vi "ResultsColumn.vi"(0 "Table Builder (Eingang)":refnum<class "Table Builder.lvclass">, 1 "Results out":T4={"Results"=[], "ResultPictures"={"Yes Ctl Refnum"=refnum, "No Ctl Refnum"=refnum}, "use Pictures"=FALSE, "Image Scale (%)"=100.0, "Autoscale? (T)"=TRUE, "Horizontal Align"=3, "Position"=0} {"Position" items=["First", "Last"]; "Horizontal Align" items=["Center", "Justified", "JustifiedAll", "Left", "Right"]}, 2 "empty?":bool, 3 "Font (Eingang)":refnum<class "Font.lvclass">, 5 "Row Formatting in":refnum<class "Formatting.lvclass">[](array[class]), 9 "Horizontal Align":i32, 11 "Fehler (Eingang, kein Fehler)":errorcluster, 12 "Result Cell Configuration":T1 {"Cell Defaults"."Vertical Align" items=["Bottom", "Middle", "Top"]; "Cell Defaults"."Horizontal Align" items=["Center", "Justified", "JustifiedAll", "Left", "Right"]}, 13 "BackgroundColor":u32, 14 "RowIndex":i32) -> (4 "Table Builder (Ausgang)":refnum<class "Table Builder.lvclass">, 6 "Row Formatting Array out":refnum<class "Formatting.lvclass">[](array[class]), 15 "Fehler (Ausgang)":errorcluster)   [LabVIEW 2020, in "PDF Interface.lvlib" / "PDF Interface Helper.lvlib"]
uses:
  PDF Interface Helper.lvlib
  <vilib>/Simplicity AI/SAI_PDF_API/Classes/Table Formatting/Formatting.lvclass
  <vilib>/Simplicity AI/SAI_PDF_API/Classes/Font/Font.lvclass
  PDFResults.ctl
  PDFResultPictures.ctl
  <vilib>/Simplicity AI/SAI_PDF_API/Classes/Table Builder/Controls/SAI_PDF_Cell Configuration.ctl
  <vilib>/Simplicity AI/SAI_PDF_API/Classes/Table Builder/Controls/SAI_PDF_Default Cell Format.ctl
  <vilib>/Simplicity AI/SAI_PDF_API/Classes/Table Builder/Controls/SAI_PDF_BorderLine.ctl
  <vilib>/Simplicity AI/SAI_PDF_API/Classes/Table Builder/Table Builder.lvclass
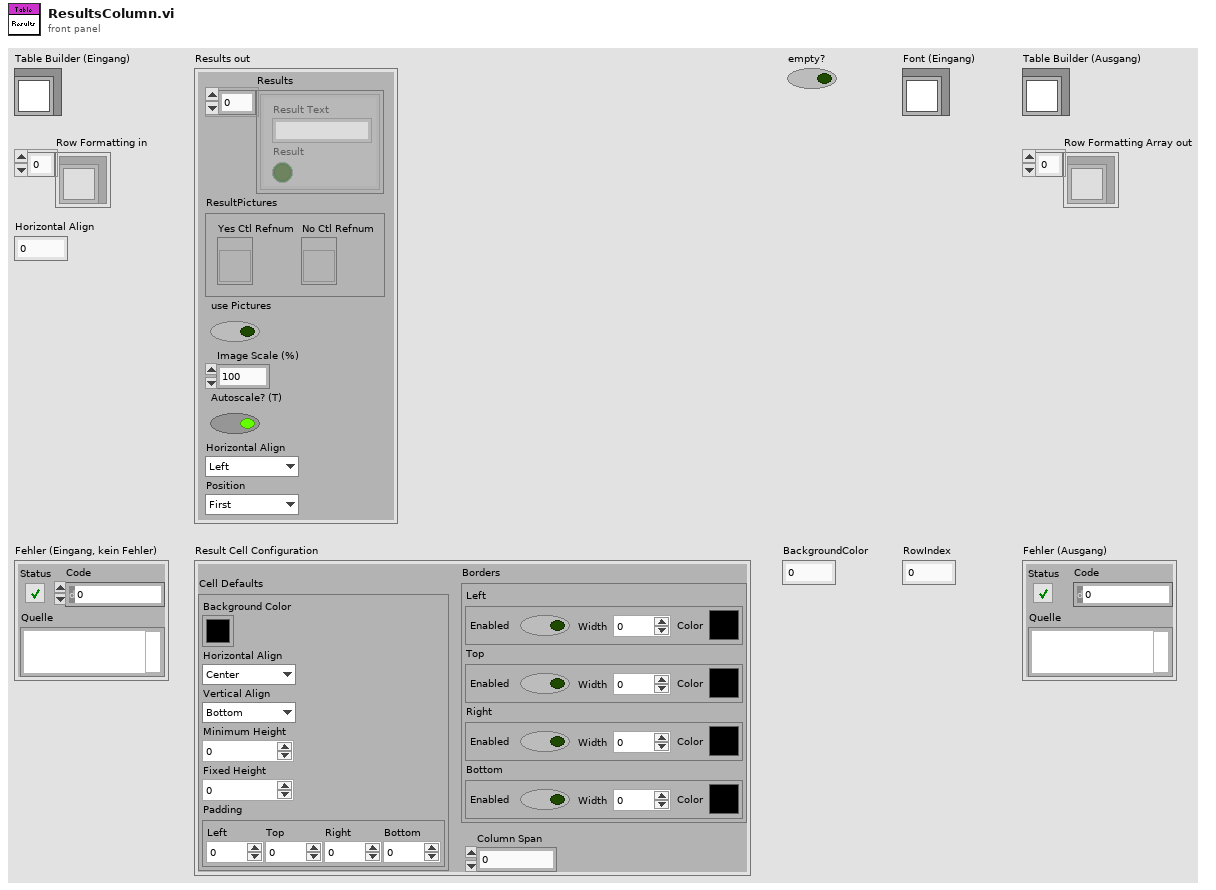
[diagram p1: front panel]
types:
  T1 = typedef "SAI_PDF_Toolkit.lvlib/Table Builder.lvclass/SAI_PDF_Cell Configuration.ctl" = cluster{"Cell Defaults":T2, "Borders":cluster{"Left":T3, "Top":T3, "Right":T3, "Bottom":T3}, "Column Span":i32}
  T2 = typedef "SAI_PDF_Toolkit.lvlib/Table Builder.lvclass/SAI_PDF_Default Cell Format.ctl" = cluster{"Background Color":u32, "Horizontal Align":i32, "Vertical Align":i32, "Minimum Height":sgl, "Fixed Height":sgl, "Padding":cluster{"Left":sgl, "Top":sgl, "Right":sgl, "Bottom":sgl}}
  T3 = typedef "SAI_PDF_Toolkit.lvlib/Table Builder.lvclass/SAI_PDF_BorderLine.ctl" = cluster{"Enabled":bool, "Width":sgl, "Color":u32}
  T4 = typedef "PDF Interface.lvlib/PDF Interface Helper.lvlib/PDFResults.ctl" = cluster{"Results":cluster{"Result Text":string, "Result":bool}[], "ResultPictures":T5, "use Pictures":bool, "Image Scale (%)":sgl, "Autoscale? (T)":bool, "Horizontal Align":i32, "Position":i32}
  T5 = typedef "PDF Interface.lvlib/PDF Interface Helper.lvlib/PDFResultPictures.ctl" = cluster{"Yes Ctl Refnum":refnum<vi>, "No Ctl Refnum":refnum<vi>}
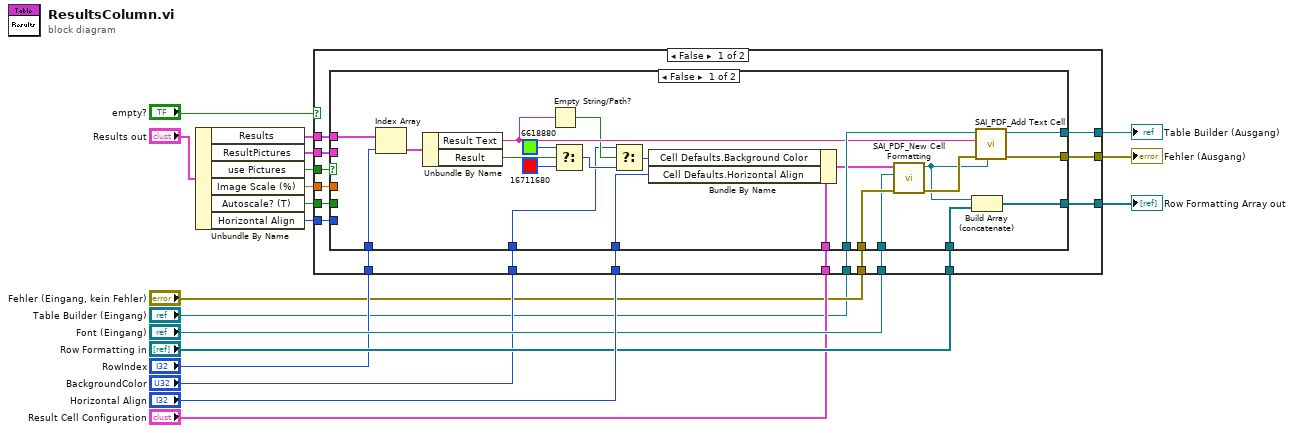
[diagram p0: block diagram]
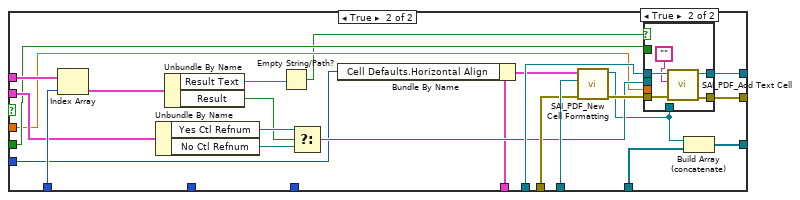
[diagram p2: hidden frame]
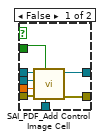
[diagram p3: hidden frame]
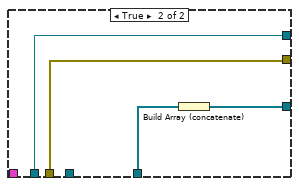
[diagram p4: hidden frame]
diagram:
  n1 = Unbundle By Name("Results out") -> ("Results"=w6:cluster{"Result Text":string, "Result":bool}[], "ResultPictures"=w4:T5, "use Pictures"=w5:bool, "Image Scale (%)"=w1:sgl, "Autoscale? (T)"=w2:bool, "Horizontal Align"=w3:i32)
  n2 = case shown="False" "empty?" {
    tunnel: "Table Builder (Eingang)" -> [w36 w100]
    tunnel: [w35 w100] -> w8
    tunnel: "Fehler (Eingang, kein Fehler)" -> [w34 w99]
    tunnel: "Font (Eingang)" -> [w33 _]
    tunnel: "Result Cell Configuration" -> [w24 _]
    tunnel: "Row Formatting in" -> [w26 w98]
    tunnel: [w27 w97] -> w19
    tunnel: [w32 w99] -> w11
    tunnel: w6 -> [w31 _]
    tunnel: "RowIndex" -> [w30 _]
    tunnel: "BackgroundColor" -> [w29 _]
    tunnel: "Horizontal Align" -> [w28 _]
    tunnel: w5 -> [w25 _]
    tunnel: w4 -> [w23 _]
    tunnel: w3 -> [w22 _]
    tunnel: w2 -> [w21 _]
    tunnel: w1 -> [w20 _]
    frame False {
      n3 = case shown="False" w25 {
        tunnel: w36 -> [w59 w80]
        tunnel: [w58 w71] -> w35
        tunnel: w34 -> [w56 w82]
        tunnel: w33 -> [w55 w83]
        tunnel: [w52 w70] -> w32
        tunnel: w31 -> [w48 w78]
        tunnel: w30 -> [w46 w77]
        tunnel: w29 -> [w42 _]
        tunnel: w28 -> [w40 _]
        tunnel: [w38 w67] -> w27
        tunnel: w26 -> [w37 w68]
        tunnel: w24 -> [w54 w66]
        tunnel: w23 -> [_ w76]
        tunnel: w22 -> [_ w64]
        tunnel: w21 -> [_ w63]
        tunnel: w20 -> [_ w62]
        frame False {
          n4 = Index Array(array=w48, index=w46) -> (element=w47:cluster{"Result Text":string, "Result":bool})
          n5 = Unbundle By Name(w47) -> ("Result Text"=w45:string, "Result"=w49:bool)
          n6 = Empty String/Path?(string/path=w45) -> (empty?=w44:bool)
          n7 = Select(t=u32 6618880 ("Color Box"), s=w49, f=u32 16711680 ("Color Box")) -> (s? t:f=w43:u32)
          n8 = Select(t=w42, s=w44, f=w43) -> (s? t:f=w41:u32)
          n9 = Bundle By Name(cluster=w54, "Cell Defaults.Background Color"=w41, "Cell Defaults.Horizontal Align"=w40) -> (w53:T1)
          n10 = call <vilib>:"SAI_PDF_New Cell Formatting.vi"("error in"=w56, "Font In"=w55, "Cell Configuration"=w53) -> ("error out"=w57:errorcluster, "Cell Formatting"=w39:refnum<class "Formatting.lvclass">)  [unwired: 7 out]
          n11 = Build Array (concatenate)(w39, w37) -> (w38:refnum<class "Formatting.lvclass">[])
          n12 = call <vilib>:"SAI_PDF_Add Text Cell.vi"("Formatting In"=w39, "error in"=w57, "Text"=w45, "Table Builder In"=w59) -> ("error out"=w52:errorcluster, "Table Builder Out"=w58:refnum<class "Table Builder.lvclass">)  [unwired: 6 out]
        }
        frame True {
          n13 = Index Array(array=w78, index=w77) -> (element=w79:cluster{"Result Text":string, "Result":bool})
          n14 = Unbundle By Name(w76) -> ("Yes Ctl Refnum"=w75:refnum<vi>, "No Ctl Refnum"=w74:refnum<vi>)
          n15 = Unbundle By Name(w79) -> ("Result Text"=w61:string, "Result"=w73:bool)
          n16 = Empty String/Path?(string/path=w61) -> (empty?=w60:bool)
          n17 = Select(t=w75, s=w73, f=w74) -> (s? t:f=w72:refnum<vi>)
          n18 = Bundle By Name(cluster=w66, "Cell Defaults.Horizontal Align"=w64) -> (w65:T1)
          n19 = call <vilib>:"SAI_PDF_New Cell Formatting.vi"("error in"=w82, "Font In"=w83, "Cell Configuration"=w65) -> ("error out"=w81:errorcluster, "Cell Formatting"=w69:refnum<class "Formatting.lvclass">)  [unwired: 7 out]
          n20 = case shown="True" w60 {
            tunnel: w81 -> [w91 w95]
            tunnel: w80 -> [w90 w96]
            tunnel: w72 -> [w89 _]
            tunnel: [w88 w94] -> w71
            tunnel: [w87 w93] -> w70
            tunnel: w69 -> [w86 _]
            tunnel: w63 -> [w85 _]
            tunnel: w62 -> [w84 _]
            frame False {
              n21 = call <vilib>:"SAI_PDF_Add Control Image Cell.vi"("Formatting In"=w86, "Autoscale? (T)"=w85, "error in"=w91, "Image Scale (%)"=w84, "Ctl Refnum In"=w89, "Table Builder In"=w90) -> ("error out"=w87:errorcluster, "Table Builder Out"=w88:refnum<class "Table Builder.lvclass">)  [unwired: 4 in]
            }
            frame True {
              n22 = call <vilib>:"SAI_PDF_Add Text Cell.vi"("error in"=w95, "Text"="", "Table Builder In"=w96) -> ("error out"=w93:errorcluster, "Table Builder Out"=w94:refnum<class "Table Builder.lvclass">)  [unwired: 1 in, 6 out]
            }
          }
          n23 = Build Array (concatenate)(w69, w68) -> (w67:refnum<class "Formatting.lvclass">[])
        }
      }
    }
    frame True {
      n24 = Build Array (concatenate)(w98) -> (w97:refnum<class "Formatting.lvclass">[])
    }
  }
  "Row Formatting Array out" <- w19
  "Fehler (Ausgang)" <- w11
  "Table Builder (Ausgang)" <- w8
